vi "Traffic Control project ( Labview and Arduino ).vi"() -> ()   [LabVIEW 2019]
uses:
  <vilib>/LabVIEW Interface for Arduino/Type Defs/Connection Type.ctl
  <vilib>/LabVIEW Interface for Arduino/Type Defs/Pin Mode.ctl
  <vilib>/LabVIEW Interface for Arduino/LabVIEW Interface for Arduino.lvlib
panel:
  in  "stop":bool
  in  "VISA resource":refnum<visa-resource-name>
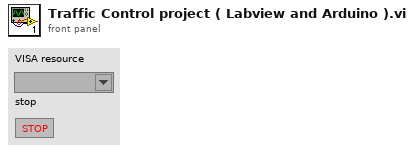
[diagram p1: front panel]
types:
  T1 = typedef "LabVIEW Interface for Arduino.lvlib/Pin Mode.ctl" = enum8{"Input", "Output"}
  T2 = typedef "LabVIEW Interface for Arduino.lvlib/Connection Type.ctl" = enum8{"USB / Serial", "XBEE", "BlueSmirf (Bluetooth)"}
  T3 = typedef "LabVIEW Interface for Arduino.lvlib/Arduino Resource.ctl" = cluster{"VISA resource":refnum<visa-resource-name>, "Board Type":T4, "Connection Type":enum8{"USB / Serial"}, "Bytes Per Packet (15)":u8}
  T4 = typedef "LabVIEW Interface for Arduino.lvlib/Board Type.ctl" = enum16{"Uno", "Dimuelanove w/Atmega 328", "Mega 2560"}
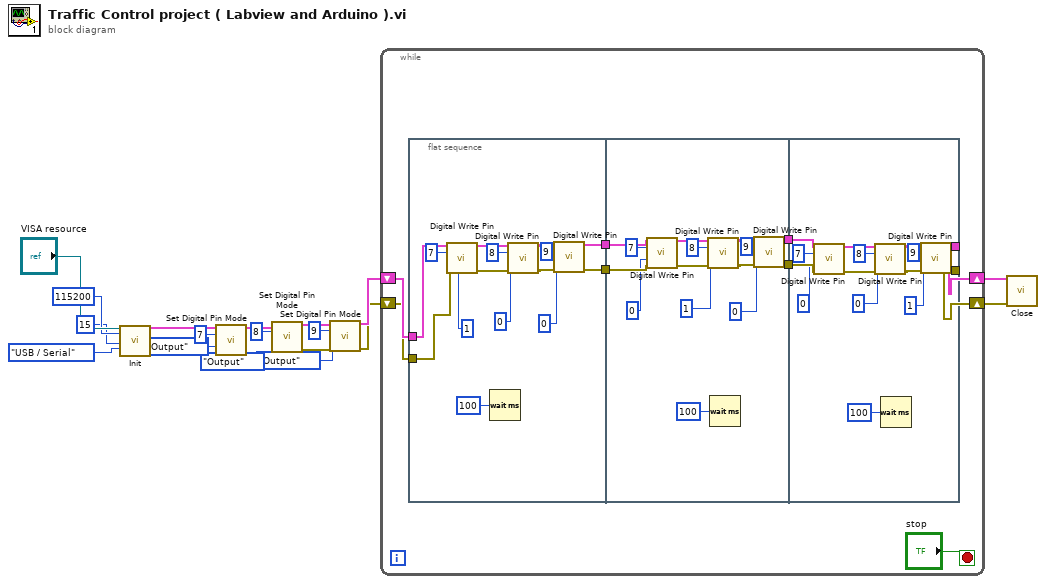
[diagram p0: block diagram]
diagram:
  n1 = call <vilib>:"Init.vi"("VISA resource"="VISA resource", "Baud Rate (115200)"=u32 115200, "Bytes Per Packet (15)"=u32 15, "Connection Type (USB/Serial)"=Connection_Type."USB / Serial") -> ("Arduino Resource"=w11:T3, "error out"=w12:errorcluster)  [unwired: 14 in]
  n2 = call <vilib>:"Set Digital Pin Mode.vi"("Arduino Resource"=w11, "Digital I/O Pin"=u8 7, "Pin Mode (Input)"=Pin_Mode."Output", "error in"=w12) -> ("Arduino Resource"=w16:T3, "error out"=w15:errorcluster)  [unwired: 10 in]
  n3 = call <vilib>:"Set Digital Pin Mode.vi"("Arduino Resource"=w16, "Digital I/O Pin"=u8 8, "Pin Mode (Input)"=Pin_Mode."Output", "error in"=w15) -> ("Arduino Resource"=w14:T3, "error out"=w13:errorcluster)  [unwired: 10 in]
  n4 = call <vilib>:"Set Digital Pin Mode.vi"("Arduino Resource"=w14, "Digital I/O Pin"=u8 9, "Pin Mode (Input)"=Pin_Mode."Output", "error in"=w13) -> ("Arduino Resource"=w4:T3, "error out"=w3:errorcluster)  [unwired: 10 in]
  n5 = while {
    shift-right: [w23] -> w2
    shift-left: w4 -> [w25]
    shift-right: [w22] -> w1
    shift-left: w3 -> [w24]
    stop <- "stop" stop-if-true
    n6 = flat-sequence {
      tunnel: w25 -> [w40]
      tunnel: w24 -> [w39]
      tunnel: [w35] -> w29
      tunnel: [w34] -> w28
      tunnel: w29 -> [w52]
      tunnel: w28 -> [w51]
      tunnel: [w50] -> w27
      tunnel: [w49] -> w26
      tunnel: w27 -> [w67]
      tunnel: w26 -> [w66]
      tunnel: [w61] -> w23
      tunnel: [w60] -> w22
      frame #0 {
        n7 = call <vilib>:"Digital Write Pin.vi"("Arduino Resource"=w40, "Digital I/O Pin (0)"=u8 7, "Value (0)"=u8 1, "error in"=w39) -> ("Arduino Resource"=w44:T3, "error out"=w43:errorcluster)  [unwired: 10 in]
        n8 = Wait (ms)(milliseconds to wait=u32 100) -> ()  [unwired: 1 out]
        n9 = call <vilib>:"Digital Write Pin.vi"("Arduino Resource"=w44, "Digital I/O Pin (0)"=u8 8, "Value (0)"=u8 0, "error in"=w43) -> ("Arduino Resource"=w42:T3, "error out"=w41:errorcluster)  [unwired: 10 in]
        n10 = call <vilib>:"Digital Write Pin.vi"("Arduino Resource"=w42, "Digital I/O Pin (0)"=u8 9, "Value (0)"=u8 0, "error in"=w41) -> ("Arduino Resource"=w35:T3, "error out"=w34:errorcluster)  [unwired: 10 in]
      }
      frame #1 {
        n11 = call <vilib>:"Digital Write Pin.vi"("Arduino Resource"=w52, "Digital I/O Pin (0)"=u8 7, "Value (0)"=u8 0, "error in"=w51) -> ("Arduino Resource"=w59:T3, "error out"=w58:errorcluster)  [unwired: 10 in]
        n12 = call <vilib>:"Digital Write Pin.vi"("Arduino Resource"=w59, "Digital I/O Pin (0)"=u8 8, "Value (0)"=u8 1, "error in"=w58) -> ("Arduino Resource"=w57:T3, "error out"=w56:errorcluster)  [unwired: 10 in]
        n13 = Wait (ms)(milliseconds to wait=u32 100) -> ()  [unwired: 1 out]
        n14 = call <vilib>:"Digital Write Pin.vi"("Arduino Resource"=w57, "Digital I/O Pin (0)"=u8 9, "Value (0)"=u8 0, "error in"=w56) -> ("Arduino Resource"=w50:T3, "error out"=w49:errorcluster)  [unwired: 10 in]
      }
      frame #2 {
        n15 = call <vilib>:"Digital Write Pin.vi"("Arduino Resource"=w67, "Digital I/O Pin (0)"=u8 7, "Value (0)"=u8 0, "error in"=w66) -> ("Arduino Resource"=w74:T3, "error out"=w73:errorcluster)  [unwired: 10 in]
        n16 = call <vilib>:"Digital Write Pin.vi"("Arduino Resource"=w74, "Digital I/O Pin (0)"=u8 8, "Value (0)"=u8 0, "error in"=w73) -> ("Arduino Resource"=w72:T3, "error out"=w71:errorcluster)  [unwired: 10 in]
        n17 = Wait (ms)(milliseconds to wait=u32 100) -> ()  [unwired: 1 out]
        n18 = call <vilib>:"Digital Write Pin.vi"("Arduino Resource"=w72, "Digital I/O Pin (0)"=u8 9, "Value (0)"=u8 1, "error in"=w71) -> ("Arduino Resource"=w61:T3, "error out"=w60:errorcluster)  [unwired: 10 in]
      }
    }
  }
  n19 = call <vilib>:"Close.vi"("Arduino Resource"=w2, "error in"=w1) -> ()  [unwired: 13 in, 1 out]
